vi "Add Channel.vi"(7 "Highlight? (F)":bool, 8 "error in":errorcluster, 9 "Channel":T1, 10 "Name":string, 11 "Parent Ref":T3 format="%.0x") -> (0 "error out":errorcluster, 3 "Channel Ref out":T3 format="%.0x")   [LabVIEW 2020, in "Communication Bus Template Scripting.lvlib"]
uses:
  <vilib>/NI VeriStand/Custom Device API/Custom Device Item Ref.ctl
  Shared/Constants.vi
  Communication Bus Template Scripting.lvlib
  Shared/Communication Bus Template Shared.lvlib
  <vilib>/NI VeriStand/Custom Device API/Custom Device API.lvlib
  <vilib>/NI VeriStand/Custom Device API/Custom Device Channel Type.ctl
  <vilib>/NI VeriStand/Custom Device API/Custom Device Channel.ctl
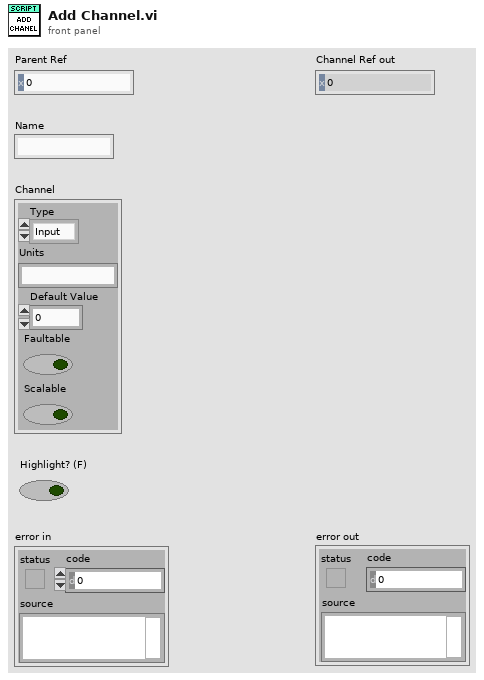
[diagram p1: front panel]
types:
  T1 = typedef "Custom Device API.lvlib/Custom Device Channel.ctl" = cluster{"Type":T2, "Units":string, "Default Value":dbl, "Faultable":bool, "Scalable":bool}
  T2 = typedef "Custom Device API.lvlib/Custom Device Channel Type.ctl" = enum16{"Input", "Output"}
  T3 = typedef "Custom Device API.lvlib/Custom Device Item Ref.ctl" = u64
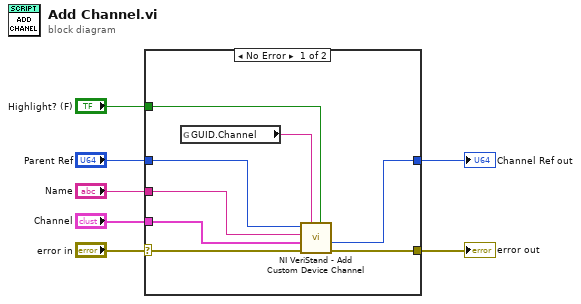
[diagram p0: block diagram]
diagram:
  n1 = case shown="No Error" "error in" {
    selector: "error in" -> [w15 w16]
    tunnel: [w14 w16] -> w6
    tunnel: "Parent Ref" -> [w11 _]
    tunnel: [w10 _] -> w4
    tunnel: "Name" -> [w12 _]
    tunnel: "Channel" -> [w9 _]
    tunnel: "Highlight? (F)" -> [w8 _]
    frame No Error {
      n2 = global read "Constants.vi" "GUID.Channel"() -> (w13:string)
      n3 = call <vilib>:"NI VeriStand - Add Custom Device Channel.vi"("Highlight? (F)"=w8, "GUID (Default Channel)"=w13, "error in (no error)"=w15, "Channel"=w9, "Channel Name"=w12, "Parent Ref in"=w11) -> ("error out"=w14:errorcluster, "Channel Ref"=w10:T3)  [unwired: 2 in, 2 out]
    }
    frame Error {
    }
  }
  "Channel Ref out" <- w4
  "error out" <- w6
